vi "PeakDetector.vi"() -> ()   [LabVIEW 2014]
doc: "This computer program created for analizing array of datafiles (*.txt) for detect peaks in current measurement range"
uses:
  User Interface/Control 1.ctl
panel:
  in  "show":bool
  out "out_cl":T1 {"max" format="%#.2g"; "min" format="%#.2g"; "start" format="%#.2g"; "delta" format="%#.2g"}
  in  "Sel":bool
  out "ReportF":path caption="Текущий файл отчета"
  out "Portion":dbl[](graph)
  out "Current DataF":path caption="Текущий файл данных"
  out "Graph":dbl[](graph)
  in  "Quit":bool
  in  "Next":bool
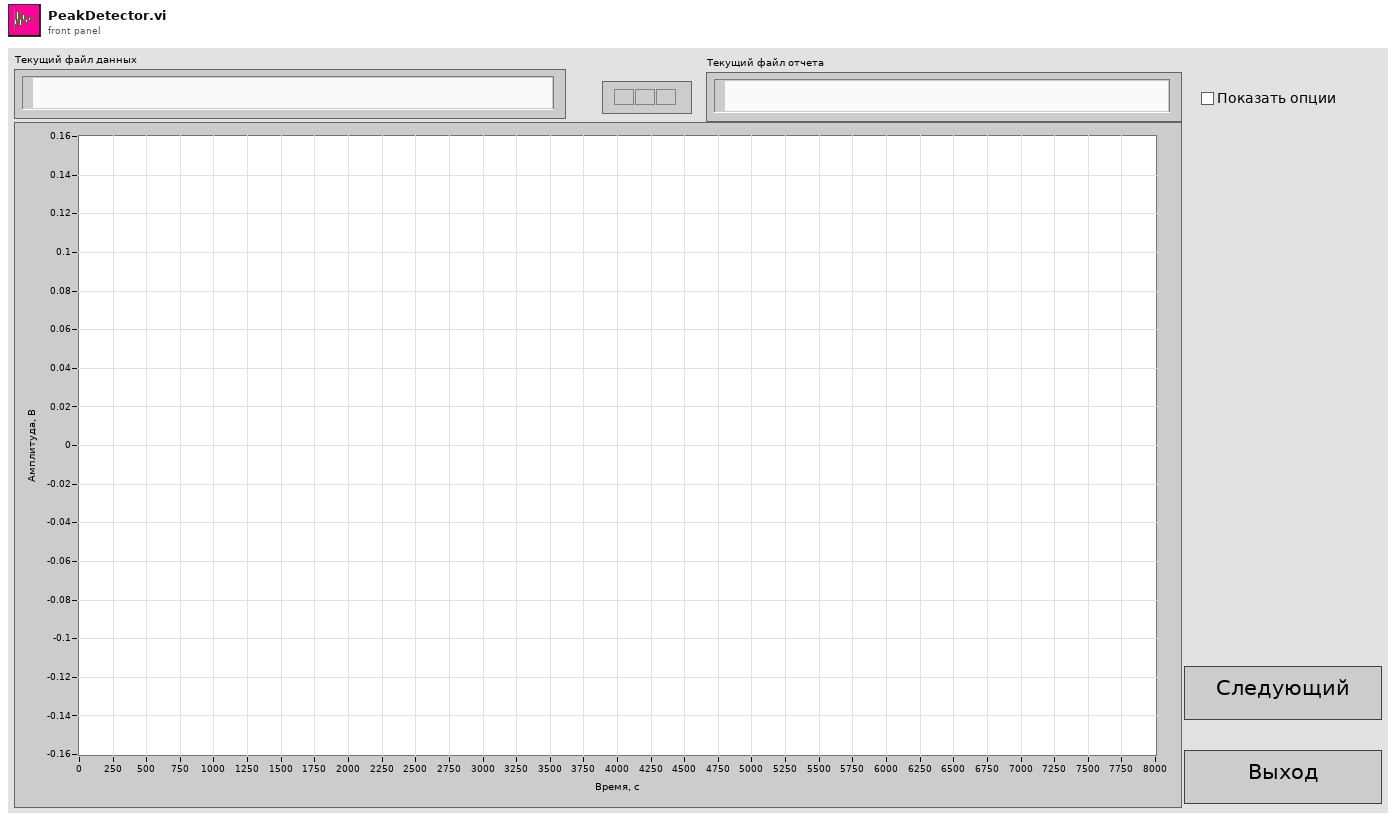
[diagram p1: front panel]
types:
  T1 = cluster{"max":dbl, "min":dbl, "start":dbl, "delta":dbl}
  T2 = enum16{"open", "open or create", "create or replace", "create", "open (read only)"}
  T3 = typedef "Control 1.ctl" = enum16{"Initialize", "Idle", "Open", "Next", "Save", "Shutdown"}
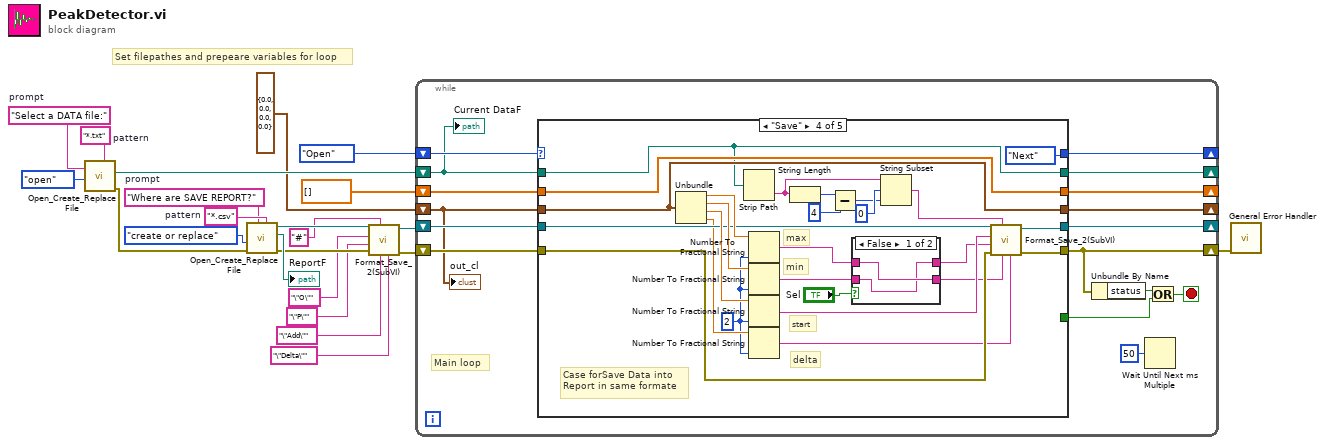
[diagram p0: block diagram]
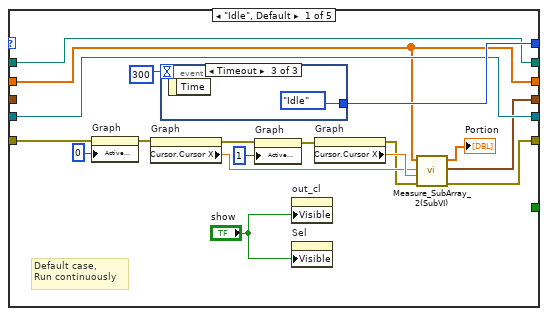
[diagram p2: hidden frame]
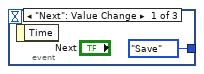
[diagram p3: hidden frame]
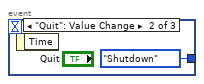
[diagram p4: hidden frame]
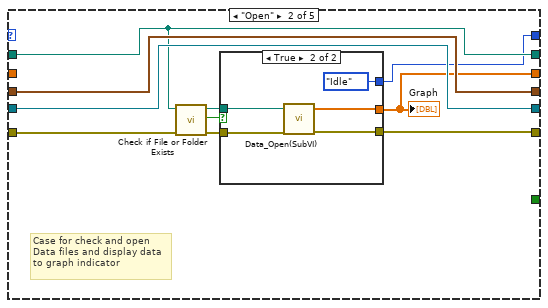
[diagram p5: hidden frame]
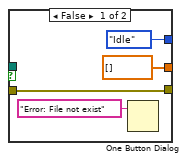
[diagram p6: hidden frame]
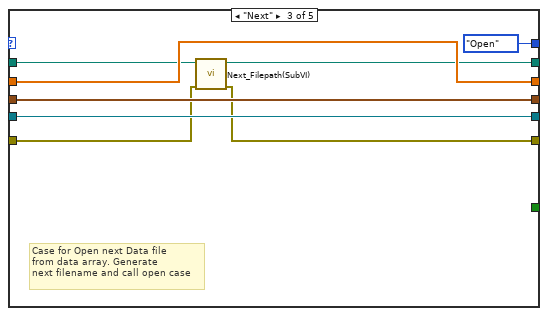
[diagram p7: hidden frame]
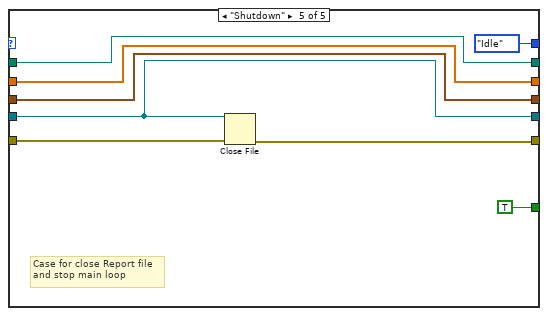
[diagram p9: hidden frame]
diagram:
  w15 = "*.csv"  # pattern
  w14 = "Where are SAVE REPORT?"  # prompt
  w16 = "*.txt"  # pattern
  w19 = "Select a DATA file:"  # prompt
  # "Set filepathes and prepeare variables for loop"
  n1 = call <vilib>:"Open_Create_Replace File.vi"("pattern"=w16, "prompt"=w19, "function (open:0)"=T2."open") -> ("error out"=w13:errorcluster, "new file path"=w18:path)  [unwired: 5 in, 2 out]
  n2 = call <vilib>:"Open_Create_Replace File.vi"("pattern"=w15, "prompt"=w14, "error in (no error)"=w13, "function (open:0)"=T2."create or replace") -> ("error out"=w10:errorcluster, "new file path"=→"ReportF":path, "refnum"=w11:refnum<file>)  [unwired: 4 in, 1 out]
  n3 = call "Format_Save_2(SubVI).vi"("5 Col"="\"Delta\"", "4 Col"="\"Add\"", "1 Col"="#", "error in (no error)"=w10, "3 Col"="\"P\"", "2 Col"="\"O\"", "refnum in"=w11) -> ("error out"=w9:errorcluster, "refnum out"=w8:refnum<file>)  [unwired: 3 in]
  n4 = while {
    shift-right: [w38] -> _
    shift-left: Control_1."Open" ("operations") -> [w37]
    shift-right: [w35] -> _
    shift-left: w18 -> [w25]
    shift-right: [w34] -> _
    shift-left: dbl[] [] -> [w33]
    shift-right: [w32] -> _
    shift-left: cluster{dbl, dbl, "Numeric Control":dbl, dbl} {0.0, 0.0, "Numeric Control"=0.0, 0.0} ("output cluster") -> [w23]
    shift-right: [w31] -> _
    shift-left: w8 -> [w30]
    shift-right: [w24] -> w20
    shift-left: w9 -> [w29]
    stop <- w26 stop-if-true
    # "Main loop"
    n5 = case shown="\"Save\"" w37 {
      tunnel: [_ _ _ _ TRUE] -> w27
      tunnel: [w56 w60 Control_1."Open" ("operations") Control_1."Next" ("operations") Control_1."Idle" ("operations")] -> w38
      tunnel: w25 -> [w55 w66 w84 w109 w123]
      tunnel: [w55 w66 w79 w109 w123] -> w35
      tunnel: [w43 w62 w85 w112 w117] -> w34
      tunnel: w33 -> [w43 _ w85 w112 w117]
      tunnel: [w44 w69 w83 w110 w122] -> w32
      tunnel: w23 -> [_ w69 w83 w110 w122]
      tunnel: [w54 w68 w82 w103 w121] -> w31
      tunnel: w30 -> [w54 w68 w82 w101 w121]
      tunnel: [w45 w61 w80 w102 w119] -> w24
      tunnel: w29 -> [w48 w67 w81 w100 w120]
      frame "Idle", Default {
        # "Default case,\nRun continuously"
        n6 = property on="Graph" class="WFGraph (strict)"(error in=w48, "Active Cursor"=u32 0) -> (error out=w50:errorcluster)  [unwired: 1 in, 1 out]
        n7 = property on="Graph" class="WFGraph (strict)"(error in=w50) -> (error out=w51:errorcluster, "Cursor.Cursor X"=w41:dbl)  [unwired: 1 in, 1 out]
        n8 = event shown="[2] Timeout" {
          selector: _ -> [_ _ _]
          dyn-events: _ -> [_ _ _]
          timeout: 300 -> [_ _ _]
          tunnel: [Control_1."Save" ("operations") Control_1."Shutdown" ("operations") Control_1."Idle" ("operations")] -> w56
          event "Next": Value Change {
            n9 = event-data() -> ()  [unwired: 1 in, 1 out]
          }
          event "Quit": Value Change {
            n10 = event-data() -> ()  [unwired: 1 in, 1 out]
          }
          event Timeout {
            n11 = event-data() -> ()  [unwired: 1 in, 1 out]
          }
        }
        n12 = property on="Graph" class="WFGraph (strict)"(error in=w51, "Active Cursor"=u32 1) -> (error out=w53:errorcluster)  [unwired: 1 in, 1 out]
        n13 = property on="out_cl" class="Clust (strict)"("Visible"="show") -> ()  [unwired: 2 in, 2 out]
        n14 = property on="Sel" class="Bool (strict)"("Visible"="show") -> ()  [unwired: 2 in, 2 out]
        n15 = property on="Graph" class="WFGraph (strict)"(error in=w53) -> (error out=w40:errorcluster, "Cursor.Cursor X"=w42:dbl)  [unwired: 1 in, 1 out]
        n16 = call "Measure_SubArray_2(SubVI).vi"("error in (no error)"=w40, "FinalPos"=w42, "StartPos"=w41, "InArray"=w43) -> ("error out"=w45:errorcluster, "output cluster"=w44:cluster{dbl, dbl, "Numeric Control":dbl, dbl}, "OutSubArray"=→"Portion":dbl[])  [unwired: 5 in]
      }
      frame "Open" {
        # "Case for check and open\nData files and display data\nto graph indicator"
        n17 = call <vilib>:"Check if File or Folder Exists.vi"("error in (no error)"=w67, "path"=w66) -> ("error out"=w64:errorcluster, "file or folder exists?"=w65:bool, "dup path"=w63:path)  [unwired: 7 in]
        n18 = case shown="True" w65 {
          tunnel: w64 -> [w73 w77]
          tunnel: w63 -> [_ w78]
          tunnel: [dbl[] [] w76] -> w62
          tunnel: [w73 w75] -> w61
          tunnel: [Control_1."Idle" ("operations") Control_1."Idle" ("operations")] -> w60
          frame False {
            n19 = One Button Dialog(message="Error: File not exist") -> ()  [unwired: 1 in, 1 out]
          }
          frame True {
            n20 = call "Data_Open(SubVI).vi"("error in (no error)"=w77, "DataFilePath"=w78) -> ("error out"=w75:errorcluster, "DataArray"=w76:dbl[])  [unwired: 8 in]
          }
        }
        "Graph" <- w62
      }
      frame "Next" {
        # "Case for Open next Data file \nfrom data array. Generate \nnext filename and call open case"
        n21 = call "Next_Filepath(SubVI).vi"("error in (no error)"=w81, "Input filepath"=w84) -> ("error out"=w80:errorcluster, "Next  filepath"=w79:path)  [unwired: 8 in]
      }
      frame "Save" {
        w88 = 2
        # "Case forSave Data into \nReport in same formate"
        # "delta"
        # "min"
        # "start"
        # "max"
        n22 = Unbundle(w110) -> (w108:dbl, w107:dbl, "Numeric Control"=w106:dbl, w89:dbl)
        n23 = Strip Path(path=w109) -> (name=w91:string)  [unwired: 1 out]
        n24 = Number To Fractional String(number=w108, precision (6)=w88) -> (F-format string=w96:string)  [unwired: 2 in]
        n25 = Number To Fractional String(number=w107, precision (6)=w88) -> (F-format string=w104:string)  [unwired: 2 in]
        n26 = Number To Fractional String(number=w106, precision (6)=w88) -> (F-format string=w99:string)  [unwired: 2 in]
        n27 = Number To Fractional String(number=w89, precision (6)=w88) -> (F-format string=w87:string)  [unwired: 2 in]
        n28 = String Length(string=w91) -> (length=w92:i32)
        n29 = Subtract(x=w92, y=4) -> (x-y=w94:i32)
        n30 = case shown="False" "Sel" {
          tunnel: w96 -> [w114 w116]
          tunnel: w104 -> [w113 w115]
          tunnel: [w113 w116] -> w98
          tunnel: [w114 w115] -> w97
          frame False {
          }
          frame True {
          }
        }
        n31 = String Subset(string=w91, offset (0)=0 ("y"), length (rest)=w94) -> (substring=w90:string)
        n32 = call "Format_Save_2(SubVI).vi"("5 Col"=w87, "4 Col"=w97, "1 Col"=w90, "error in (no error)"=w100, "3 Col"=w98, "2 Col"=w99, "refnum in"=w101) -> ("error out"=w102:errorcluster, "refnum out"=w103:refnum<file>)  [unwired: 3 in]
      }
      frame "Shutdown" {
        # "Case for close Report file\nand stop main loop"
        n33 = Close File(refnum=w121, error in=w120) -> (error out=w119:errorcluster)  [unwired: 1 out]
      }
    }
    n34 = Unbundle By Name(w24) -> ("status"=w28:bool)
    n35 = Wait Until Next ms Multiple(millisecond multiple=u32 50) -> ()  [unwired: 1 out]
    n36 = Or(x=w28, y=w27) -> (x .or. y?=w26:bool)
    "Current DataF" <- w25
    "out_cl" <- w23
  }
  n37 = call <vilib>:"General Error Handler.vi"("error in (no error)"=w20) -> ()  [unwired: 10 in, 5 out]
